vi "MatchPos2RECT (SubVI).vi"(11 "Match element":T1) -> (3 "Rectangle":cluster{"x":sgl, "y":sgl, dbl, dbl})   [LabVIEW 2016]
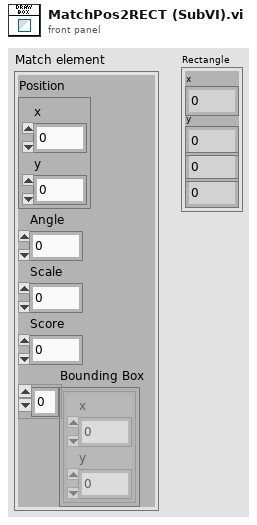
[diagram p1: front panel]
types:
  T1 = cluster{"Position":cluster{"x":sgl, "y":sgl}, "Angle":sgl, "Scale":sgl, "Score":sgl, "Bounding Box":cluster{"x":sgl, "y":sgl}[]}
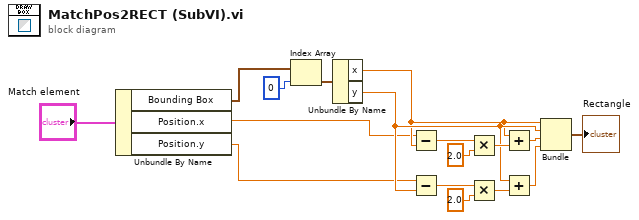
[diagram p0: block diagram]
diagram:
  n1 = Unbundle By Name("Match element") -> ("Bounding Box"=w3:cluster{"x":sgl, "y":sgl}[], "Position.x"=w2:sgl, "Position.y"=w1:sgl)
  n2 = Index Array(array=w3, index=0) -> (element=w6:cluster{"x":sgl, "y":sgl})
  n3 = Unbundle By Name(w6) -> ("x"=w10:sgl, "y"=w11:sgl)
  n4 = Subtract(x=w2, y=w10) -> (x-y=w14:sgl)
  n5 = Subtract(x=w1, y=w11) -> (x-y=w16:sgl)
  n6 = Multiply(x=w14, y=2.0) -> (x*y=w15:dbl)
  n7 = Multiply(x=w16, y=2.0) -> (x*y=w17:dbl)
  n8 = Add(x=w10, y=w15) -> (x+y=w8:dbl)
  n9 = Add(x=w11, y=w17) -> (x+y=w9:dbl)
  n10 = Bundle("x"=w10, "y"=w11, w8, w9) -> (→"Rectangle":cluster{"x":sgl, "y":sgl, dbl, dbl})  [unwired: 1 in]
